vi "Test gRPC cRIO.vi"(11 "Test Case In":refnum<class "Test Virtual NEO480.lvclass">) -> (0 "error out":errorcluster, 3 "Test Case Out":refnum<class "Test Virtual NEO480.lvclass">)   [LabVIEW 2024, in "Test Virtual NEO480.lvclass"]
uses:
  Test Virtual NEO480.lvclass
  C:/Program Files/National Instruments/LabVIEW 2025/vi.lib/Astemes/LUnit/Test Case.lvclass
  Source/Configure Strategies/gRPC XNET Read Raw CAN Frame Strategy/gRPC XNET Read Raw CAN Frame Strategy.lvclass
  D:/git/HAL/Source/Interfaces/IConfigure/IConfigure.lvclass
  Source/Virtual NEO480/Virtual NEO480.lvclass
  Source/Config from JSON/Config from JSON.lvclass
  D:/git/HAL/Source/Interfaces/IConfiguration/IConfiguration.lvclass
  Source/DBC Communicator/DBC Communicator.lvclass
  D:/git/HAL/Source/Interfaces/IInstrument/IInstrument.lvclass
  <vilib>/Astemes/LUnit/Test Case.lvclass/Test Case.ctl
  <vilib>/Astemes/LUnit/Append Pass Result.vi
  <vilib>/Astemes/LUnit/Append Fail Result.vi
  <vilib>/Astemes/LUnit/Run In UI.vi
  <vilib>/Utility/error.llb/Clear Errors.vi
  <vilib>/Astemes/LUnit/Test Case.lvclass
panel:
  in  "stop":bool
  out "Time Stamp":timestamp format="%<%x %.3X>T"
  out "Temperature":dbl
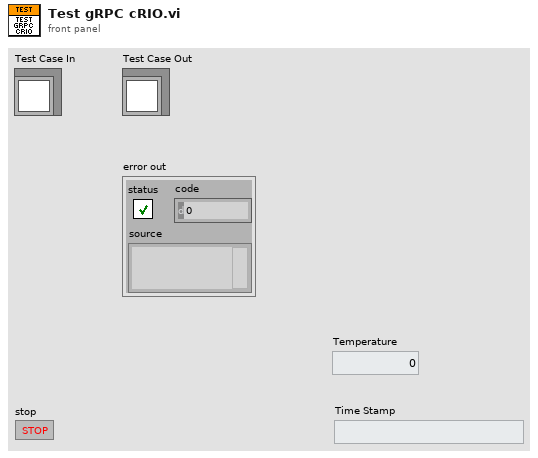
[diagram p1: front panel]
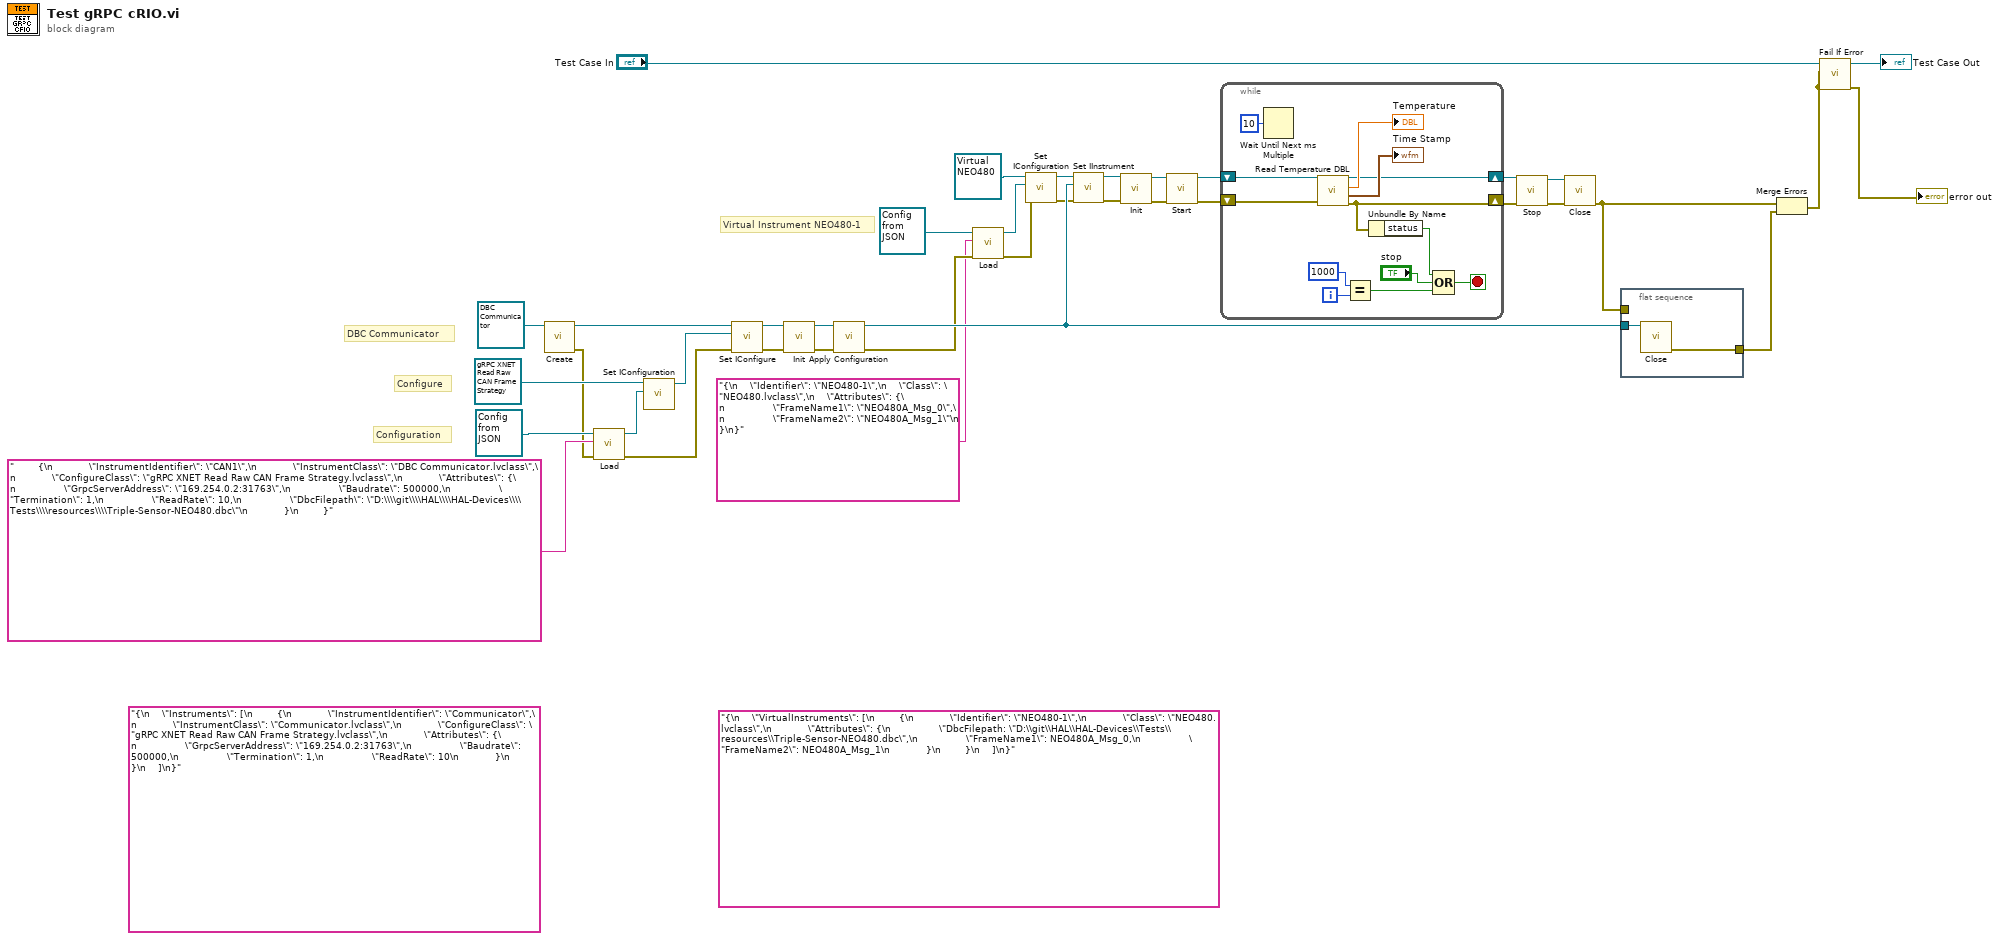
[diagram p0: block diagram]
diagram:
  (unwired) "{\n    \"VirtualInstruments\": [\n        {\n            \"Identifier\": \"NEO480-1\",\n            \"Class\": \"NEO480.lvclass\",\n            \"Attributes\": {\n                \"DbcFilepath: \"D:\\git\\HAL\\HAL-Devices\\Tests\\resources\\Triple-Sensor-NEO480.dbc\",\n                \"FrameName1\": NEO480A_Msg_0,\n                \"FrameName2\": NEO480A_Msg_1\n            }\n        }\n    ]\n}"
  (unwired) "{\n    \"Instruments\": [\n        {\n            \"InstrumentIdentifier\": \"Communicator\",\n            \"InstrumentClass\": \"Communicator.lvclass\",\n            \"ConfigureClass\": \"gRPC XNET Read Raw CAN Frame Strategy.lvclass\",\n            \"Attributes\": {\n                \"GrpcServerAddress\": \"169.254.0.2:31763\",\n                \"Baudrate\": 500000,\n                \"Termination\": 1,\n                \"ReadRate\": 10\n            }\n        }\n    ]\n}" ("Source")
  # "Virtual Instrument NEO480-1"
  # "DBC Communicator"
  # "Configure"
  # "Configuration"
  n1 = call-dynamic "Create.vi"("reference in"=refnum<class "DBC Communicator.lvclass"> refnum ("DBC Communicator")) -> ("Error Out"=w5:errorcluster, "reference out"=w30:refnum<class "DBC Communicator.lvclass">)  [unwired: 9 in]
  n2 = call-dynamic "Load.vi"("error in"=w5, "Source"="        {\n            \"InstrumentIdentifier\": \"CAN1\",\n            \"InstrumentClass\": \"DBC Communicator.lvclass\",\n            \"ConfigureClass\": \"gRPC XNET Read Raw CAN Frame Strategy.lvclass\",\n            \"Attributes\": {\n                \"GrpcServerAddress\": \"169.254.0.2:31763\",\n                \"Baudrate\": 500000,\n                \"Termination\": 1,\n                \"ReadRate\": 10,\n                \"DbcFilepath\": \"D:\\\\git\\\\HAL\\\\HAL-Devices\\\\Tests\\\\resources\\\\Triple-Sensor-NEO480.dbc\"\n            }\n        }", "Config From JSON in"=refnum<class "Config from JSON.lvclass"> refnum ("Config from JSON.lvclass")) -> ("error out"=w4:errorcluster, "Config From JSON out"=w31:refnum<class "Config from JSON.lvclass">)  [unwired: 7 in]
  n3 = call-dynamic "Set IConfiguration.vi"("IConfiguration"=w31, "gRPC XNET Read Raw CAN Frame Strategy in"=refnum<class "gRPC XNET Read Raw CAN Frame Strategy.lvclass"> refnum ("gRPC XNET Read Raw CAN Frame Strategy.lvclass")) -> ("gRPC XNET Read Raw CAN Frame Strategy out"=w6:refnum<class "gRPC XNET Read Raw CAN Frame Strategy.lvclass">)  [unwired: 9 in]
  n4 = call-dynamic "Set IConfigure.vi"("Error In"=w4, "IConfigure"=w6, "Communicator in"=w30) -> ("Error Out"=w16:errorcluster, "Communicator out"=w14:refnum<class "DBC Communicator.lvclass">)  [unwired: 7 in]
  n5 = call-dynamic "Init.vi"("Error In"=w16, "Communicator in"=w14) -> ("Error Out"=w15:errorcluster, "Communicator out"=w13:refnum<class "DBC Communicator.lvclass">)  [unwired: 8 in]
  n6 = call-dynamic "Apply Configuration.vi"("Error In"=w15, "reference in"=w13) -> ("Error Out"=w11:errorcluster, "reference out"=w12:refnum<class "DBC Communicator.lvclass">)  [unwired: 8 in]
  n7 = call-dynamic "Load.vi"("error in"=w11, "Source"="{\n    \"Identifier\": \"NEO480-1\",\n    \"Class\": \"NEO480.lvclass\",\n    \"Attributes\": {\n                \"FrameName1\": \"NEO480A_Msg_0\",\n                \"FrameName2\": \"NEO480A_Msg_1\"\n    }\n}", "Config From JSON in"=refnum<class "Config from JSON.lvclass"> refnum ("Config from JSON.lvclass")) -> ("error out"=w2:errorcluster, "Config From JSON out"=w27:refnum<class "Config from JSON.lvclass">)  [unwired: 7 in]
  n8 = call-dynamic "Set IConfiguration.vi"("IConfiguration"=w27, "NEO480 in"=refnum<class "Virtual NEO480.lvclass"> refnum ("NEO480.lvclass")) -> ("NEO480 out"=w26:refnum<class "Virtual NEO480.lvclass">)  [unwired: 8 in, 1 out]
  n9 = call-dynamic "Set IInstrument.vi"("error in"=w2, "IInstrument"=w12, "NEO480 in"=w26) -> ("error out"=w3:errorcluster, "NEO480 out"=w23:refnum<class "Virtual NEO480.lvclass">)  [unwired: 7 in]
  n10 = call-dynamic "Init.vi"("error in"=w3, "NEO480 in"=w23) -> ("error out"=w18:errorcluster, "NEO480 out"=w25:refnum<class "Virtual NEO480.lvclass">)  [unwired: 8 in]
  n11 = call-dynamic "Start.vi"("error in"=w18, "NEO480 in"=w25) -> ("error out"=w17:errorcluster, "NEO480 out"=w24:refnum<class "Virtual NEO480.lvclass">)  [unwired: 8 in]
  n12 = while {
    shift-right: [w39] -> w21
    shift-left: w24 -> [w48]
    shift-right: [w40] -> w22
    shift-left: w17 -> [w38]
    i -> [w45]
    stop <- w46 stop-if-true
    n13 = Wait Until Next ms Multiple(millisecond multiple=u32 10) -> ()  [unwired: 1 out]
    n14 = call-dynamic "Read Temperature DBL.vi"("error in"=w38, "NEO480 in"=w48) -> ("error out"=w40:errorcluster, "Time Stamp"=→"Time Stamp":timestamp, "Temperature"=→"Temperature":dbl, "NEO480 out"=w39:refnum<class "Virtual NEO480.lvclass">)  [unwired: 6 in]
    n15 = Equal?(x=1000, y=w45) -> (x = y?=w42:bool)
    n16 = Unbundle By Name(w40) -> ("status"=w41:bool)
    n17 = Compound Arithmetic op=OR(w41, "stop", w42) -> (w46:bool)
  }
  n18 = call-dynamic "Stop.vi"("error in"=w22, "NEO480 in"=w21) -> ("error out"=w20:errorcluster, "NEO480 out"=w19:refnum<class "Virtual NEO480.lvclass">)  [unwired: 8 in]
  n19 = call-dynamic "Close.vi"("error in"=w20, "NEO480 in"=w19) -> ("error out"=w10:errorcluster)  [unwired: 8 in, 1 out]
  n20 = flat-sequence {
    tunnel: w12 -> [w52]
    tunnel: w10 -> [_]
    tunnel: [w51] -> w8
    frame #0 {
      n21 = call-dynamic "Close.vi"("reference in"=w52) -> ("Error Out"=w51:errorcluster)  [unwired: 9 in, 1 out]
    }
  }
  n22 = Merge Errors(w10, w8) -> (w9:errorcluster)
  n23 = call <vilib>:"Fail If Error.vi"("error in (no error)"=w9, "Assert error"=w9, "LUnit Test Case In"="Test Case In") -> ("error out"=→"error out":errorcluster, "LUnit Test Case Out"=→"Test Case Out":refnum<class "Test Virtual NEO480.lvclass">)  [unwired: 7 in]
